vi "test_Bitfile Reload_DMA.vi"(8 "error in (no error)":errorcluster, 11 "TestCase in":refnum<class "FPGA Addon Bitfile Reload Unit Tests.lvclass">=refnum) -> (0 "error out":errorcluster, 3 "TestCase out":refnum<class "FPGA Addon Bitfile Reload Unit Tests.lvclass">)   [LabVIEW 2026, in "FPGA Addon Bitfile Reload Unit Tests.lvclass"]
uses:
  FPGA Addon Bitfile Reload Unit Tests.lvclass
  Addon/Addon Shared/Types/DMA Information.ctl
  Addon/Addon Shared/FPGA Addon Shared.lvlib
  FPGA Addon Test Class/FPGA Addon Test Class.lvclass
  APIs/Scripting API/Scripting API.lvlib
  Addon/Addon System Explorer/FPGA Addon System Explorer.lvlib
  Addon/Addon Shared/Types/Delacing Scheme.ctl
  Addon/Addon Shared/Types/DMA Acquisition Mode.ctl
  Addon/Addon Shared/Types/DMA Settings.ctl
  Addon/Addon Shared/Types/FPGA Addon Data Type.ctl
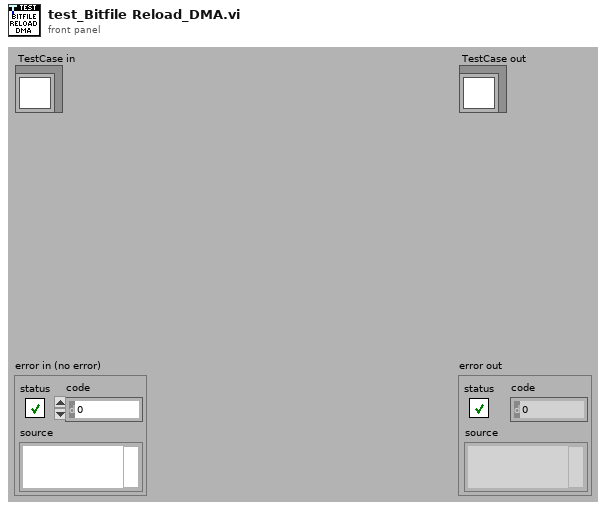
[diagram p1: front panel]
types:
  T1 = typedef "FPGA Addon Shared.lvlib/DMA Settings.ctl" = cluster{"Number of Channels":u8, "Delacing Scheme":T2, "Update Rate":u32, "dt":dbl, "Mode":T3, "Number of Samples":u32, "DMA Host Buffer":u32}
  T2 = typedef "FPGA Addon Shared.lvlib/Delacing Scheme.ctl" = enum8{"Interleaved", "Bitpacked"}
  T3 = typedef "FPGA Addon Shared.lvlib/DMA Acquisition Mode.ctl" = enum8{"Continuous", "Triggered Finite"}
  T4 = typedef "FPGA Addon Shared.lvlib/DMA Information.ctl" = cluster{"Name":string, "Data Type":T5}
  T5 = typedef "FPGA Addon Shared.lvlib/FPGA Addon Data Type.ctl" = enum8{"<Null>", "I8", "I16", "I32", "I64", "U8", "U16", "U32", "U64", "SGL", "Boolean", "Analog PWM In Settings", "Analog PWM In", "Digital PWM In Settings", "Digital PWM In", "Digital PWM Out", "Sine Out", "FXP", "FXP+/-24.5", "FXP+/-16.5", "FXP+/-32.8", "FXP+/-64.32", "FXP+/-16.7", "FXP+/-20.5", "FXP+/-27.5", "FXP+/-32.16", "FXP+16.3", "FXP+18.3", "Digital Static In", "Digital Static Out", "Digital Static In Settings", "Digital WSS Out", "Quad Encoder Settings", "Quad Encoder In", "Group"}
  T6 = typedef "Custom Device API.lvlib/Custom Device Item Ref.ctl" = u64
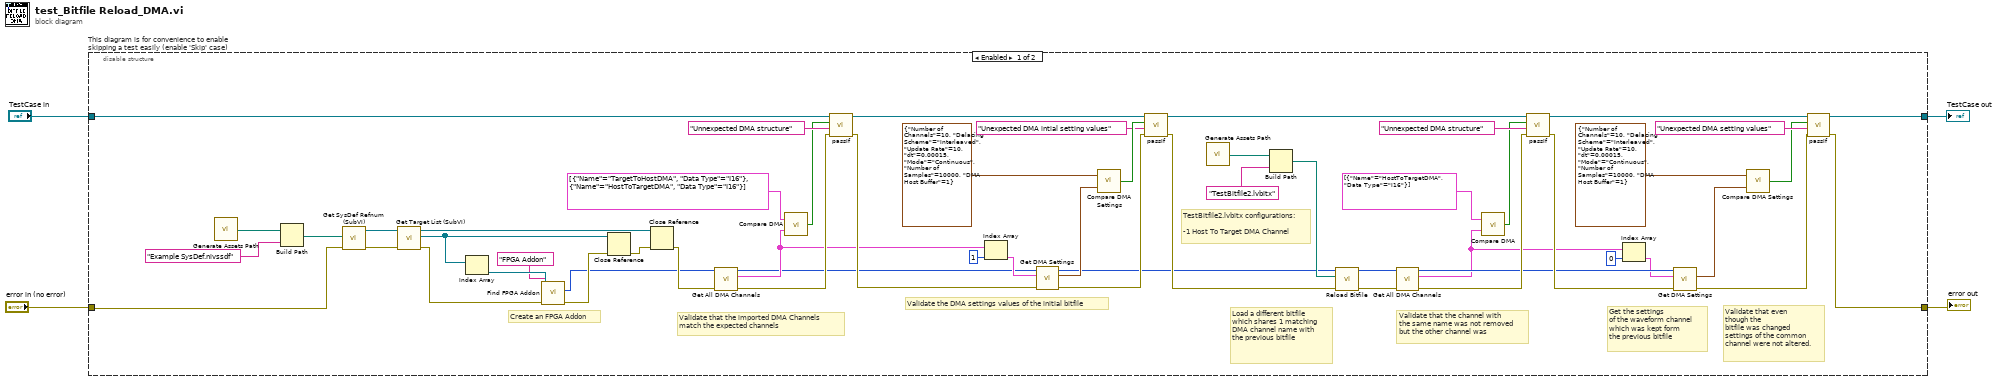
[diagram p0: block diagram]
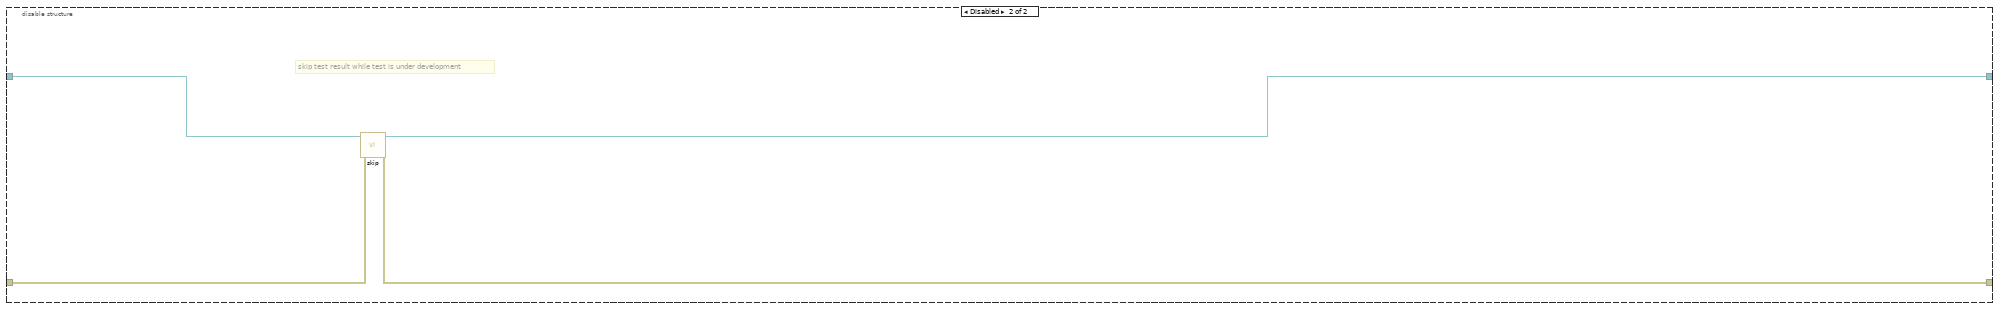
[diagram p2: hidden frame]
diagram:
  n1 = disable-structure "This diagram is for convenience to enable skipping a test easily (enable 'Skip' case)" shown="Enabled" {
    disable-tunnel: "TestCase in" -> [w35 w64]
    disable-tunnel: [w25 w62] -> w1
    disable-tunnel: [w26 w63] -> w3
    disable-tunnel: "error in (no error)" -> [w34 w61]
    frame Enabled {
      # "Validate the DMA settings values of the initial bitfile"
      # "Validate that even \nthough the \nbitfile was changed\nsettings of the common \nchannel were not altered."
      # "Get the settings \nof the waveform channel\nwhich was kept form \nthe previous bitfile"
      # "TestBitfile2.lvbitx configurations:\n\n-1 Host To Target DMA Channel"
      # "Validate that the channel with \nthe same name was not removed\nbut the other channel was"
      # "Load a different bitfile\nwhich shares 1 matching\nDMA channel name with \nthe previous bitfile"
      # "Validate that the imported DMA Channels \nmatch the expected channels"
      # "Create an FPGA Addon"
      n2 = call "Generate Assets Path.vi"() -> ("Assets path"=w52:path)
      n3 = Build Path(base path=w52, name or relative path="Example SysDef.nivssdf") -> (appended path=w59:path)
      n4 = call "Get SysDef Refnum (SubVI).vi"("error in (no error)"=w34, "System Definition path"=w59) -> ("error out"=w57:errorcluster, "NationalInstruments.VeriStand.SystemDefinitionAPI.SystemDefinition"=w58:refnum<k39>)  [unwired: 8 in]
      n5 = call "Get Target List (SubVI).vi"("error in (no error)"=w57, "NationalInstruments.VeriStand.SystemDefinitionAPI.SystemDefinition"=w58) -> ("error out"=w47:errorcluster, "Target List Refnums"=w56:refnum<k39>[], "NationalInstruments.VeriStand.SystemDefinitionAPI.SystemDefinition"=w55:refnum<k39>)  [unwired: 7 in]
      n6 = Index Array(array=w56) -> (element=w45:refnum<k39>)  [unwired: 1 in]
      n7 = call "Find FPGA Addon.vi"("error in"=w47, "FPGA addon name"="FPGA Addon", "NationalInstruments.VeriStand.SystemDefinitionAPI.Target"=w45) -> ("error out"=w46:errorcluster, "FPGA addon refnum out"=w42:T6)  [unwired: 5 in, 2 out]
      n8 = Close Reference(reference=w56, error in (no error)=w46) -> (error out=w54:errorcluster)
      n9 = Close Reference(reference=w55, error in (no error)=w54) -> (error out=w43:errorcluster)
      n10 = call "Get All DMA Channels.vi"("error in (no error)"=w43, "FPGA addon refnum in"=w42) -> ("error out"=w41:errorcluster, "DMA channels out"=w13:T4[], "FPGA addon refnum out"=w6:T6)  [unwired: 7 in]
      n11 = call "Compare DMA.vi"("Target bitfile DMA in"=w13, "Reference bitfile DMA in"=T4[] [{"Name"="TargetToHostDMA", "Data Type"=enum."I16"}, {"Name"="HostToTargetDMA", "Data Type"=enum."I16"}] ("DMA channels out")) -> ("Equal ?"=w40:bool)
      n12 = call-dynamic "passIf.vi"("error in (no error)"=w41, "message (\"\")"="Unnexpected DMA structure" ("message (\"\")"), "pass"=w40, "TestCase in"=w35) -> ("error out"=w14:errorcluster, "TestCase out"=w18:refnum<class "FPGA Addon Bitfile Reload Unit Tests.lvclass">)  [unwired: 6 in]
      n13 = Index Array(array=w13, index=1) -> (element=w15:T4)
      n14 = call "Get DMA Settings.vi"("error in (no error)"=w14, "DMA Channel in"=w15, "FPGA addon refnum in"=w6) -> ("error out"=w8:errorcluster, "DMA Settings"=w11:T1, "FPGA addon refnum out"=w5:T6)  [unwired: 6 in]
      n15 = call "Compare DMA Settings.vi"("DMA Settings 2"=w11, "DMA Settings 1"=T1 {"Number of Channels"=10, "Delacing Scheme"=enum."Interleaved", "Update Rate"=10, "dt"=0.00015, "Mode"=enum."Continuous", "Number of Samples"=10000, "DMA Host Buffer"=1} ("DMA Settings")) -> ("equal?"=w10:bool)
      n16 = call-dynamic "passIf.vi"("error in (no error)"=w8, "message (\"\")"="Unexpected DMA intial setting values" ("message (\"\")"), "pass"=w10, "TestCase in"=w18) -> ("error out"=w7:errorcluster, "TestCase out"=w17:refnum<class "FPGA Addon Bitfile Reload Unit Tests.lvclass">)  [unwired: 6 in]
      n17 = call "Generate Assets Path.vi"() -> ("Assets path"=w50:path)
      n18 = Build Path(base path=w50, name or relative path="TestBitfile2.lvbitx") -> (appended path=w49:path)
      n19 = call "Reload Bitfile.vi"("error in (no error)"=w7, "NewVal"=w49, "Item Ref in"=w5) -> ("error out"=w39:errorcluster, "Section Ref out"=w37:T6)  [unwired: 7 in]
      n20 = call "Get All DMA Channels.vi"("error in (no error)"=w39, "FPGA addon refnum in"=w37) -> ("error out"=w38:errorcluster, "DMA channels out"=w24:T4[], "FPGA addon refnum out"=w28:T6)  [unwired: 7 in]
      n21 = call "Compare DMA.vi"("Target bitfile DMA in"=w24, "Reference bitfile DMA in"=T4[] [{"Name"="HostToTargetDMA", "Data Type"=enum."I16"}] ("DMA channels out")) -> ("Equal ?"=w36:bool)
      n22 = call-dynamic "passIf.vi"("error in (no error)"=w38, "message (\"\")"="Unnexpected DMA structure" ("message (\"\")"), "pass"=w36, "TestCase in"=w17) -> ("error out"=w30:errorcluster, "TestCase out"=w31:refnum<class "FPGA Addon Bitfile Reload Unit Tests.lvclass">)  [unwired: 6 in]
      n23 = Index Array(array=w24, index=0) -> (element=w22:T4)
      n24 = call "Get DMA Settings.vi"("error in (no error)"=w30, "DMA Channel in"=w22, "FPGA addon refnum in"=w28) -> ("error out"=w29:errorcluster, "DMA Settings"=w20:T1)  [unwired: 6 in, 1 out]
      n25 = call "Compare DMA Settings.vi"("DMA Settings 2"=w20, "DMA Settings 1"=T1 {"Number of Channels"=10, "Delacing Scheme"=enum."Interleaved", "Update Rate"=10, "dt"=0.00015, "Mode"=enum."Continuous", "Number of Samples"=10000, "DMA Host Buffer"=1} ("DMA Settings")) -> ("equal?"=w19:bool)
      n26 = call-dynamic "passIf.vi"("error in (no error)"=w29, "message (\"\")"="Unexpected DMA setting values" ("message (\"\")"), "pass"=w19, "TestCase in"=w31) -> ("error out"=w26:errorcluster, "TestCase out"=w25:refnum<class "FPGA Addon Bitfile Reload Unit Tests.lvclass">)  [unwired: 6 in]
    }
    frame Disabled {
      # "skip test result while test is under development"
      n27 = call <vilib>:"skip.vi"("error in (no error)"=w61, "TestCase in"=w64) -> ("error out"=w63:errorcluster, "TestCase out"=w62:refnum<class "FPGA Addon Bitfile Reload Unit Tests.lvclass">)  [unwired: 8 in]
    }
  }
  "error out" <- w3
  "TestCase out" <- w1
